vi "PWM.vi"() -> ()   [LabVIEW 2017]
uses:
  <vilib>/rvi/eio/common/nirviEmuTemplateMethod_errors.vi
  <vilib>/eio/EIONode/EIONode.xnode
panel:
  in  "DutyC":u32
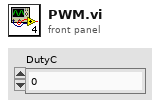
[diagram p1: front panel]
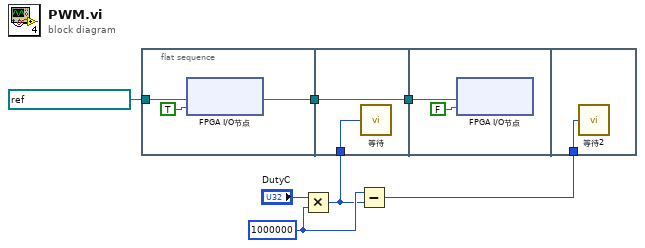
[diagram p0: block diagram]
diagram:
  w3 = u32 1000000
  n1 = flat-sequence {
    tunnel: refnum<k21> "ConnectorA/DIO8" ("FPGA I/O输入") -> [w10]
    tunnel: [w9] -> w6
    tunnel: w6 -> [w12]
    tunnel: [w12] -> w5
    tunnel: w1 -> [w11]
    tunnel: w5 -> [w14]
    tunnel: w2 -> [w15]
    frame #0 {
      n2 = xnode "FPGA I/O节点"("I/O项"=TRUE, "FPGA I/O输入"=w10) -> ("FPGA I/O输出"=w9:refnum<k21>)
    }
    frame #1 {
      n3 = call "等待"("Count(uSec)"=w11) -> ()  [unwired: 1 out]
    }
    frame #2 {
      n4 = xnode "FPGA I/O节点"("I/O项"=FALSE, "FPGA I/O输入"=w14) -> ()  [unwired: 1 out]
    }
    frame #3 {
      n5 = call "等待2"("Count(uSec)"=w15) -> ()  [unwired: 1 out]
    }
  }
  n6 = Multiply(x="DutyC", y=w3) -> (x*y=w1:u32)
  n7 = Subtract(x=w3, y=w1) -> (x-y=w2:u32)
